vi "Get Host Remote IP&Port.vi"(0 "IP:Port:Master/Slave":string) -> (2 "This instance is Master?":bool, 4 "IP":string, 5 "Port":u16)   [LabVIEW 2021, in "Utilities.lvlib"]
uses:
  Utilities.lvlib
  <vilib>/regexp/Match Regular Expression.xnode
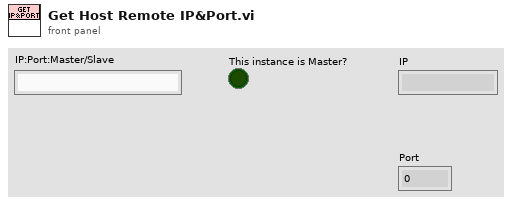
[diagram p1: front panel]
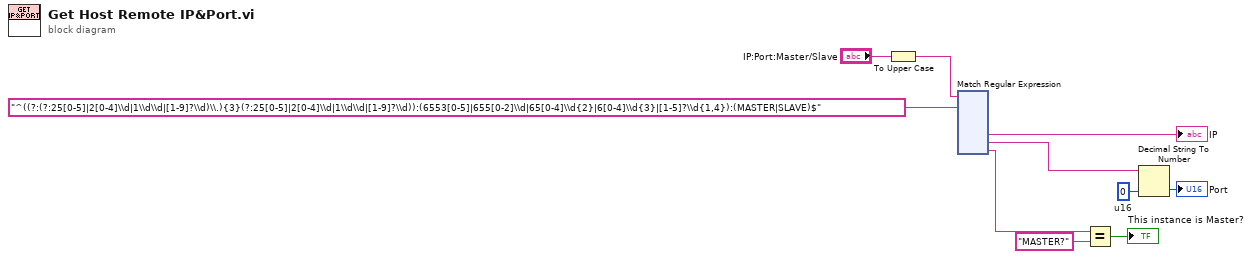
[diagram p0: block diagram]
diagram:
  w5 = u16 0  # u16
  n1 = To Upper Case(1:"IP:Port:Master/Slave") -> (0:w3:string)
  n2 = xnode "Match Regular Expression"("input string"=w3, "regular expression"="^((?:(?:25[0-5]|2[0-4]\\d|1\\d\\d|[1-9]?\\d)\\.){3}(?:25[0-5]|2[0-4]\\d|1\\d\\d|[1-9]?\\d)):(6553[0-5]|655[0-2]\\d|65[0-4]\\d{2}|6[0-4]\\d{3}|[1-5]?\\d{1,4}):(MASTER|SLAVE)$") -> ("submatch 1"=→"IP":string, "submatch 2"=w7:string, "submatch 3"=w4:string)  [unwired: 4 in, 5 out]
  n3 = Equal?(x=w4, y="MASTER?") -> (x = y?=→"This instance is Master?":bool)
  n4 = Decimal String To Number(string=w7, default (0L)=w5) -> (number=→"Port":u16)  [unwired: 1 in, 1 out]
